vi "Rotate Data By Teeth Angle.vi"(5 "CycleAngle?":T1 caption="FPGA simulation angle reference", 7 "Missing Tooth Angle":dbl, 11 "One VR Crank Period":dbl[](array[numeric])) -> (3 "Rotated to desired angle":dbl[](array[numeric]))   [LabVIEW 2011, in "Engine Sim System Explorer.lvlib"]
uses:
  Engine Sim System Explorer.lvlib
  TypeDefs/AngleReference.ctl
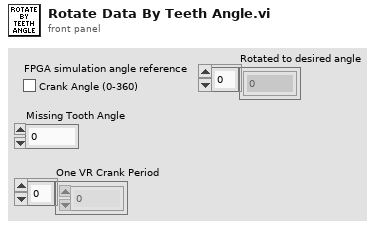
[diagram p1: front panel]
types:
  T1 = typedef "Engine Sim System Explorer.lvlib/AngleReference.ctl" = bool
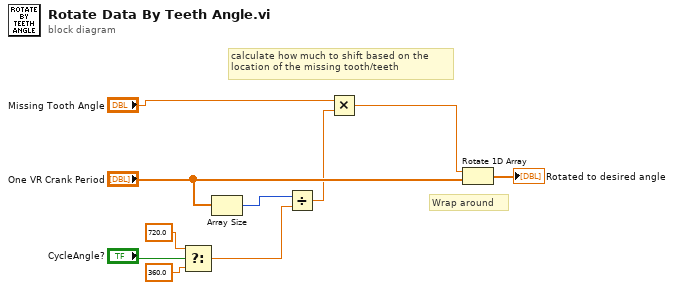
[diagram p0: block diagram]
diagram:
  # "Wrap around"
  # "calculate how much to shift based on the \nlocation of the missing tooth/teeth"
  n1 = Select(t=720.0, s="CycleAngle?", f=360.0 ("t")) -> (s? t:f=w1:dbl)
  n2 = Array Size(array="One VR Crank Period") -> (size(s)=w5:i32)
  n3 = Divide(x=w5, y=w1) -> (x/y=w7:dbl)
  n4 = Multiply(x="Missing Tooth Angle", y=w7) -> (x*y=w8:dbl)
  n5 = Rotate 1D Array(1:"One VR Crank Period", 2:w8) -> (0:→"Rotated to desired angle":dbl[])
